vi "Total Images.vi"(8 "error in (no error)":errorcluster, 10 "Total Images":u32, 11 "UserInterface in":refnum<class "UserInterface.lvclass">) -> (0 "error out":errorcluster, 3 "UserInterface out":refnum<class "UserInterface.lvclass">)   [LabVIEW 2022 SP3, in "UserInterface.lvlib" / "UserInterface.lvclass"]
uses:
  UserInterface.lvclass
  UserInterface.lvclass/UserInterface.ctl
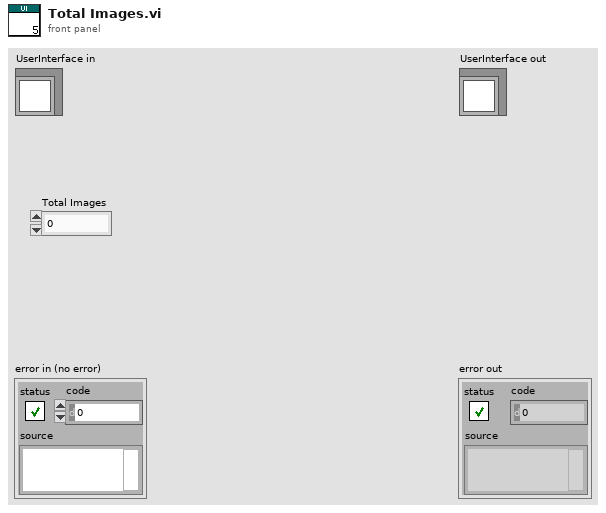
[diagram p1: front panel]
types:
  T1 = cluster{"Image List":refnum<vi>, "ProgressBar":refnum<vi>, "Log":refnum<vi>, "Image Indicator":refnum<vi>}
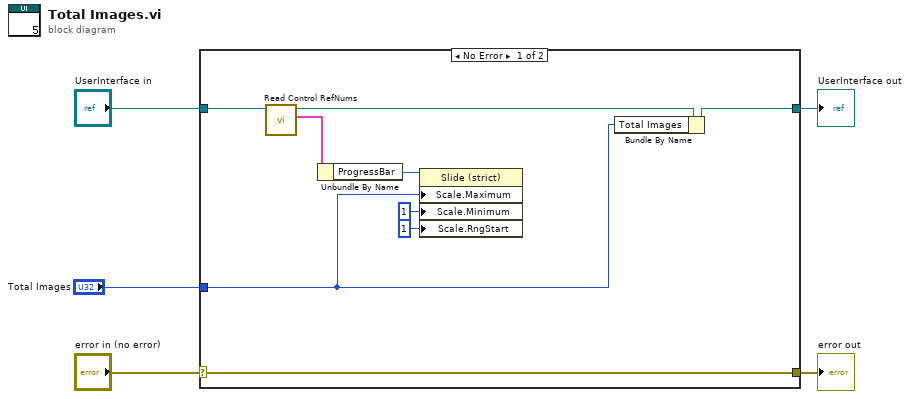
[diagram p0: block diagram]
diagram:
  n1 = case shown="No Error" "error in (no error)" {
    selector: "error in (no error)" -> [w14 w16]
    tunnel: [w14 w16] -> w4
    tunnel: [w7 w15] -> w2
    tunnel: "UserInterface in" -> [w13 w15]
    tunnel: "Total Images" -> [w6 _]
    frame No Error {
      n2 = call "Read Control RefNums.vi"("UserInterface in"=w13) -> ("Control RefNums"=w11:T1, "UserInterface out"=w12:refnum<class "UserInterface.lvclass">)  [unwired: 8 in, 1 out]
      n3 = Unbundle By Name(w11) -> ("ProgressBar"=w10:refnum<vi>)
      n4 = property class="Slide (strict)"(reference=w10, "Scale.Maximum"=w6, "Scale.Minimum"=u32 1 ("Scale.Range:Minimum"), "Scale.RngStart"=u32 1 ("Scale.Range:Start")) -> ()  [unwired: 1 in, 2 out]
      n5 = Bundle By Name(cluster=w12, "Total Images"=w6) -> (w7:refnum<class "UserInterface.lvclass">)
    }
    frame Error {
    }
  }
  "error out" <- w4
  "UserInterface out" <- w2
